vi "Launch VI.vi"(8 "Error In":errorcluster) -> (0 "Error Out":errorcluster)   [LabVIEW 2018]
doc: "This subVI lauches Stations based on a Strictly Typed VI reference. The number of Station\nVIs lauched is the number you enter on the # of Stations Control"
panel:
  # "How it works\n \nhttp://zone.ni.com/reference/en-XX/help/371361L-01/lvhowto/acbr_call_and_forget/"
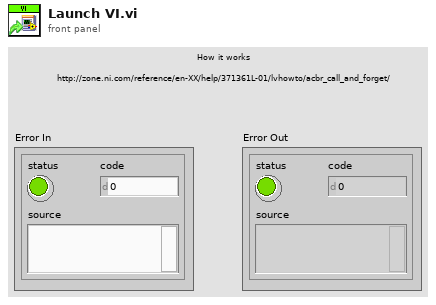
[diagram p1: front panel]
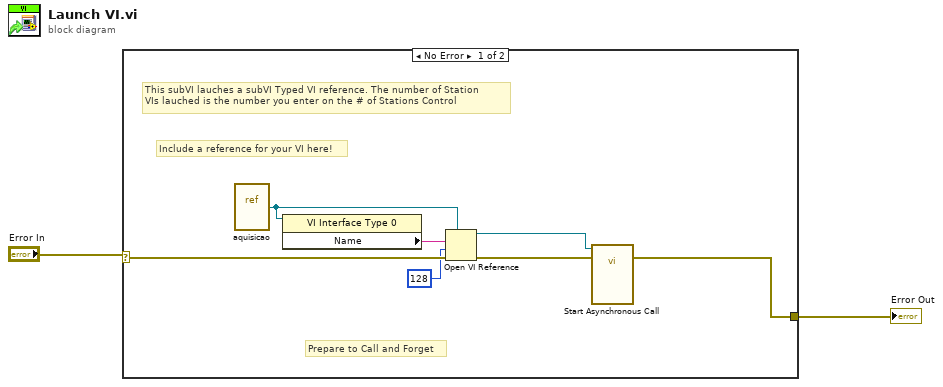
[diagram p0: block diagram]
diagram:
  n1 = case shown="No Error" "Error In" {
    selector: "Error In" -> [w8 w10]
    tunnel: [w9 w10] -> w1
    frame No Error {
      # "Include a reference for your VI here!"
      # "Prepare to Call and Forget"
      # "This subVI lauches a subVI Typed VI reference. The number of Station\nVIs lauched is the number you enter on the # of Stations Control"
      n2 = vi-ref "aquisicao.vi"() -> (w6:refnum<vi>)
      n3 = property class="VI Interface Type 0"(reference=w6) -> ("Name"=w5:string)  [unwired: 1 in, 2 out]
      n4 = Open VI Reference(type specifier VI Refnum (for type only)=w6, vi path=w5, options=128, error in (no error)=w8) -> (vi reference=w7:refnum<vi>, error out=w3:errorcluster)  [unwired: 2 in]
      n5 = call-by-ref "Start Asynchronous Call"(reference=w7, error in=w3) -> (error out=w9:errorcluster)  [unwired: 12 in, 1 out]
    }
    frame Error {
      # "In case an error is entered in this SubVI, no code is executed and the error is propagated."
    }
  }
  "Error Out" <- w1
